vi "Cmd Transaction (C).vi"(4 "error in (no error)":errorcluster, 5 "isolation level (chaos)":T1, 6 "operation (begin)":T2, 7 "command reference":T3) -> (0 "error out":errorcluster, 3 "command reference out":T3)   [LabVIEW 2020, in "NI_Database_API.lvlib"]
doc: "Begins, commits, or rolls back a transaction for any type of reference. Wire data to the reference input to determine the polymorphic instance to use or manually select the instance."
uses:
  <vilib>/addons/database/NI_Database_API.lvlib
  <vilib>/addons/database/Command.llb/Cmd ObjectReference.ctl
  <vilib>/addons/database/Auxilliary.llb/DB Tools Transaction.ctl
  <vilib>/addons/database/Auxilliary.llb/DB Tools Isolation Level.ctl
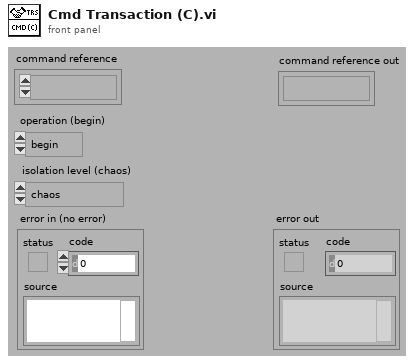
[diagram p1: front panel]
types:
  T1 = typedef "NI_Database_API.lvlib/DB Tools Isolation Level.ctl" = enum16{"chaos", "read uncommitted", "read committed", "repeatable read", "serializable"}
  T2 = typedef "NI_Database_API.lvlib/DB Tools Transaction.ctl" = enum16{"begin", "commit", "rollback"}
  T3 = typedef "NI_Database_API.lvlib/Cmd ObjectReference.ctl" = refnum<k1>
  T4 = typedef "NI_Database_API.lvlib/Cmd DataMembers.ctl" = cluster{"ADODB._Command":refnum<k7>, "Connection":T5}
  T5 = typedef "NI_Database_API.lvlib/Conn ObjectReference.ctl" = refnum<k1>
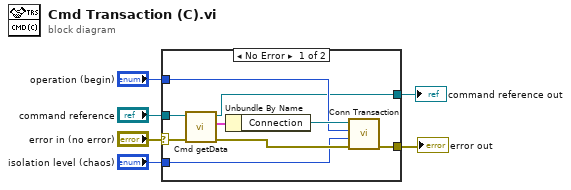
[diagram p0: block diagram]
diagram:
  n1 = case shown="No Error" "error in (no error)" {
    selector: "error in (no error)" -> [w7 w17]
    tunnel: "command reference" -> [w15 w16]
    tunnel: "operation (begin)" -> [w11 _]
    tunnel: [w10 w17] -> w4
    tunnel: [w9 w16] -> w3
    tunnel: "isolation level (chaos)" -> [w8 _]
    frame No Error {
      n2 = call <vilib>:"Cmd getData.vi"("error in (no error)"=w7, "command reference"=w15) -> ("error out"=w12:errorcluster, "data"=w14:T4, "command reference out"=w9:T3)  [unwired: 2 in, 1 out]
      n3 = Unbundle By Name(w14) -> ("Connection"=w13:T5)
      n4 = call <vilib>:"Conn Transaction.vi"("error in (no error)"=w12, "isolation level (chaos)"=w8, "operation (begin)"=w11, "connection reference"=w13) -> ("error out"=w10:errorcluster)  [unwired: 2 in, 1 out]
    }
    frame Error {
    }
  }
  "command reference out" <- w3
  "error out" <- w4
